vi "UUT modules Read Temperature and Voltages.vi"(7 "baud rate (9600)":u32=115200, 8 "error in (no error)":errorcluster, 9 "parity (0:none)":enum16{"None", "Odd", "Even", "Mark", "Space"}(ring)=enum."Odd", 10 "write buffer":string, 11 "VISA resource name":refnum<visa-resource-name>="COM10") -> (0 "error out":errorcluster, 1 "APOS_Temperature":dbl, 2 "ANEG_Voltage":dbl, 3 "DPOS_Voltage":dbl, 4 "ANEG_Temperature":dbl, 5 "APOS_Voltage":dbl, 6 "DPOS_Temperature":dbl)   [LabVIEW 2020]
uses:
  01ee9392-5957-46b9-92ae-044cd3ca9714.vi
panel:
  out "Result":string
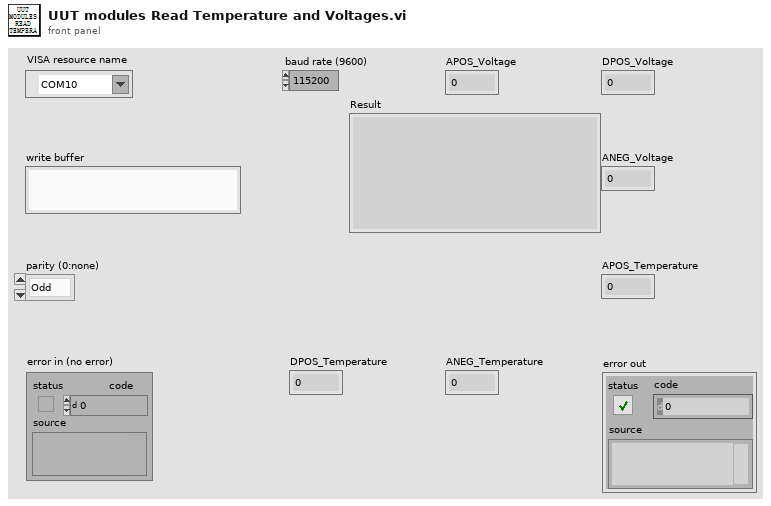
[diagram p1: front panel]
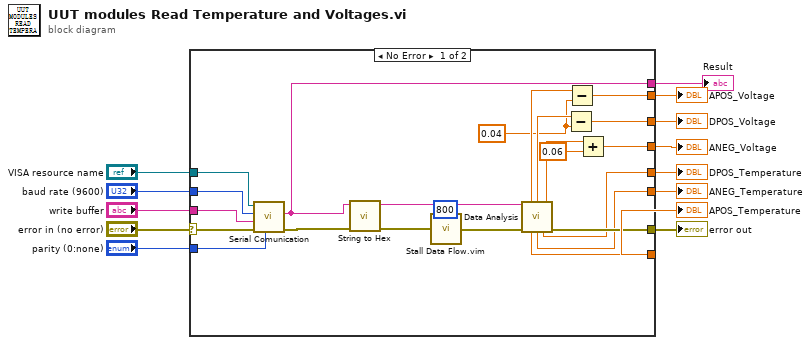
[diagram p0: block diagram]
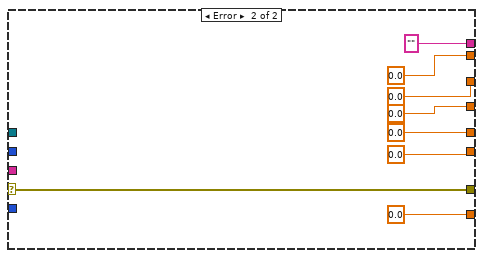
[diagram p2: hidden frame]
diagram:
  n1 = case shown="No Error" "error in (no error)" {
    selector: "error in (no error)" -> [w34 w44]
    tunnel: "VISA resource name" -> [w36 _]
    tunnel: "parity (0:none)" -> [w35 _]
    tunnel: "write buffer" -> [w33 _]
    tunnel: "baud rate (9600)" -> [w32 _]
    tunnel: [w28 w44] -> w8
    tunnel: [w27 0.0 ("DPOS_Temperature")] -> w7
    tunnel: [w26 0.0 ("ANEG_Temperature")] -> w6
    tunnel: [w25 0.0 ("APOS_Temperature")] -> w5
    tunnel: [w15 0.0 ("ANEG_Voltage")] -> w4
    tunnel: [w16 0.0 ("DPOS_Voltage")] -> w3
    tunnel: [w17 0.0 ("APOS_Voltage")] -> w2
    tunnel: [w21 "" ("Result")] -> w1
    frame No Error {
      w18 = 0.04 ("y")
      n2 = call "Serial Comunication.vi"("parity (0:none)"=w35, "error in (no error)"=w34, "write buffer"=w33, "baud rate (9600)"=w32, "VISA resource name"=w36) -> ("error out"=w31:errorcluster, "Result"=w21:string)  [unwired: 4 in, 1 out]
      n3 = call "String to Hex.vi"("error in"=w31, "Insert_String"=w21) -> ("error out"=w30:errorcluster, "Hex_String"=w29:string)  [unwired: 8 in]
      n4 = call "Stall Data Flow.vim"("value in"=w30, "milliseconds to wait"=u32 800) -> ("value out"=w20:errorcluster)  [unwired: 1 out]
      n5 = call "Data Analysis.vi"("Data In"=w29, "error in"=w20) -> ("APOS_Voltage"=w22:dbl, "DPOS_Voltage"=w23:dbl, "ANEG_Voltage"=w24:dbl, "APOS_Temperature"=w25:dbl, "ANEG_Temperature"=w26:dbl, "DPOS_Temperature"=w27:dbl, "error out"=w28:errorcluster)  [unwired: 7 in]
      n6 = Subtract(x=w23, y=w18) -> (x-y=w16:dbl)
      n7 = Subtract(x=w22, y=w18) -> (x-y=w17:dbl)
      n8 = Add(x=w24, y=0.06) -> (x+y=w15:dbl)
    }
    frame Error {
    }
  }
  "APOS_Voltage" <- w2
  "DPOS_Voltage" <- w3
  "ANEG_Voltage" <- w4
  "APOS_Temperature" <- w5
  "ANEG_Temperature" <- w6
  "DPOS_Temperature" <- w7
  "error out" <- w8
  "Result" <- w1
